vi "SingleEvent.vi"(8 "error in (no error)":errorcluster) -> (0 "error out":errorcluster, 3 "UserEvent":T1)   [LabVIEW 2017, in "TimerEngine.lvlib" / "TimerEngine.lvclass"]
uses:
  TimerEngine.lvclass
  _Typedef/Timer-UserEvent.ctl
  _Typedef/Timer-EventCluster.ctl
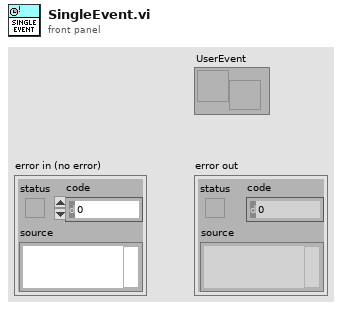
[diagram p1: front panel]
types:
  T1 = typedef "TimerEngine.lvlib/TimerEngine.lvclass/Timer-UserEvent.ctl" = refnum<user-event>
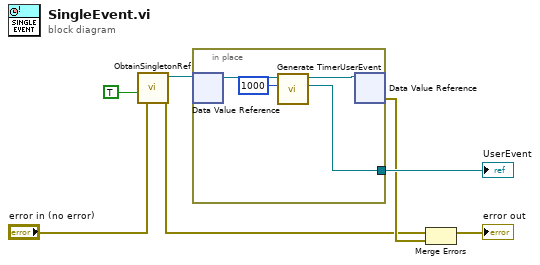
[diagram p0: block diagram]
diagram:
  n1 = call "ObtainSingletonRef.vi"("error in (no error)"="error in (no error)", "SingleEvent?(F)"=TRUE) -> ("error out"=w1:errorcluster, "data value reference"=w4:refnum<data-value>)  [unwired: 7 in, 1 out]
  n2 = in-place {
    in-place-border: [w11] -> w5
    n3 = in-place-dvr #1(w4) -> (w10:refnum<class "TimerEngine.lvclass">)  [unwired: 1 out]
    n4 = call "Generate TimerUserEvent.vi"("TimePeroid(ms)"=1000, "TimerEngine in"=w10) -> ("UserEvent"=w11:T1, "TimerEngine out"=w9:refnum<class "TimerEngine.lvclass">)  [unwired: 8 in]
    n5 = in-place-dvr #1(w9) -> (w3:errorcluster)  [unwired: 1 out]
  }
  "UserEvent" <- w5
  n6 = Merge Errors(w1, w3) -> (→"error out":errorcluster)
